vi "SetLightTower&Switch.vi"(6 "Supress Match Error (F)":bool, 8 "error in (no error)":errorcluster, 9 "UpdateValue? (F)":bool[](array[boolean]), 10 "RoomAlert Device":T1, 11 "RoomAlert in":refnum<class "RoomAlert.lvclass">) -> (0 "error out":errorcluster, 3 "RoomAlert out":refnum<class "RoomAlert.lvclass">)   [LabVIEW 2018, in "SensorPlugins.lvlib" / "RoomAlert.lvclass"]
doc: "Sets the LED and audio value of the LightTower alarm."
uses:
  RoomAlert.lvclass
  TypeDefinitions/RoomAlertControls.ctl
  RoomAlert.lvclass/RoomAlert.ctl
  <vilib>/Utility/error.llb/Error Cluster From Error Code.vi
  <vilib>/ErrorRing/Error Ring.xnode
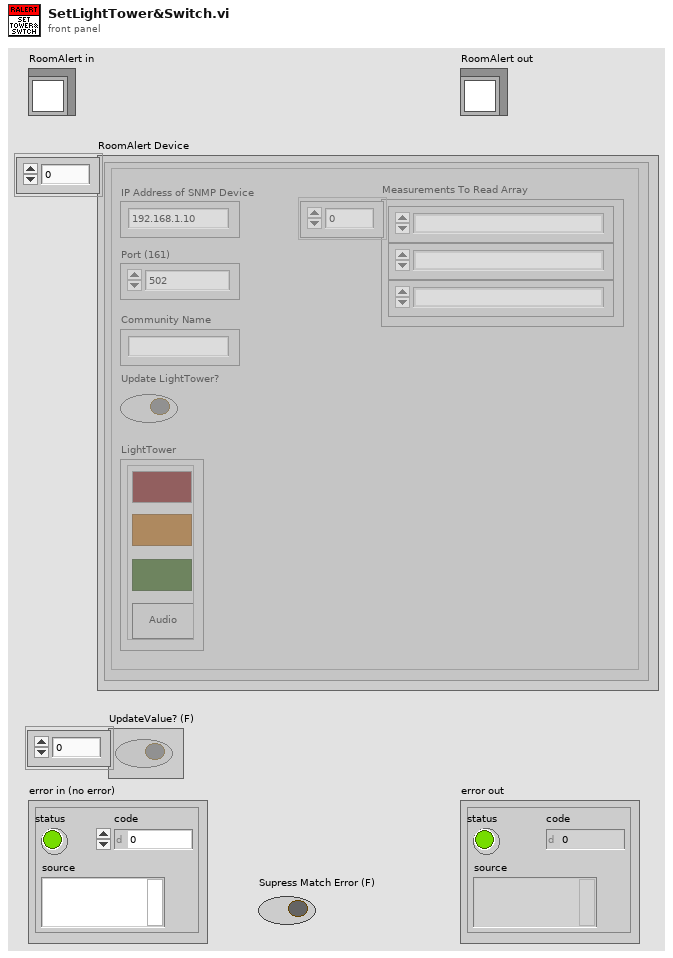
[diagram p1: front panel]
types:
  T1 = typedef "SensorPlugins.lvlib/RoomAlert.lvclass/RoomAlertControls.ctl" = cluster{"Connected?":bool, "IP Address of SNMP Device":string, "Port (161)":u16, "Community Name":string, "Measurements To Read Array":u16[], "Update LightTower?":bool, "LightTower":cluster{"Red":bool, "Amber":bool, "Green":bool, "Audio":bool}, "RoomAlert Model ID":string, "Sensor OID Numbers":string[][], "Sensor Light Tower OID Numbers":string[][]}[]
  T2 = typedef "SensorPlugins.lvlib/RoomAlert.lvclass/MeasurementControls.ctl" = cluster{"Measurement RefreshTime (ms)":u32, "Measurement Name":string, "Timeout(ms)":i32, "Amber Warning Light Configuration":cluster{"Warning Temperture (Degrees C)":dbl, "Temperature Delta (Degrees C/Minute)":dbl, "Time Window (Minutes)":dbl}}
  T3 = cluster{"Red":bool, "Amber":bool, "Green":bool, "Audio":bool}
  T4 = typedef "SensorPlugins.lvlib/RoomAlert.lvclass/CommunicationControls.ctl" = refnum<k16>[]
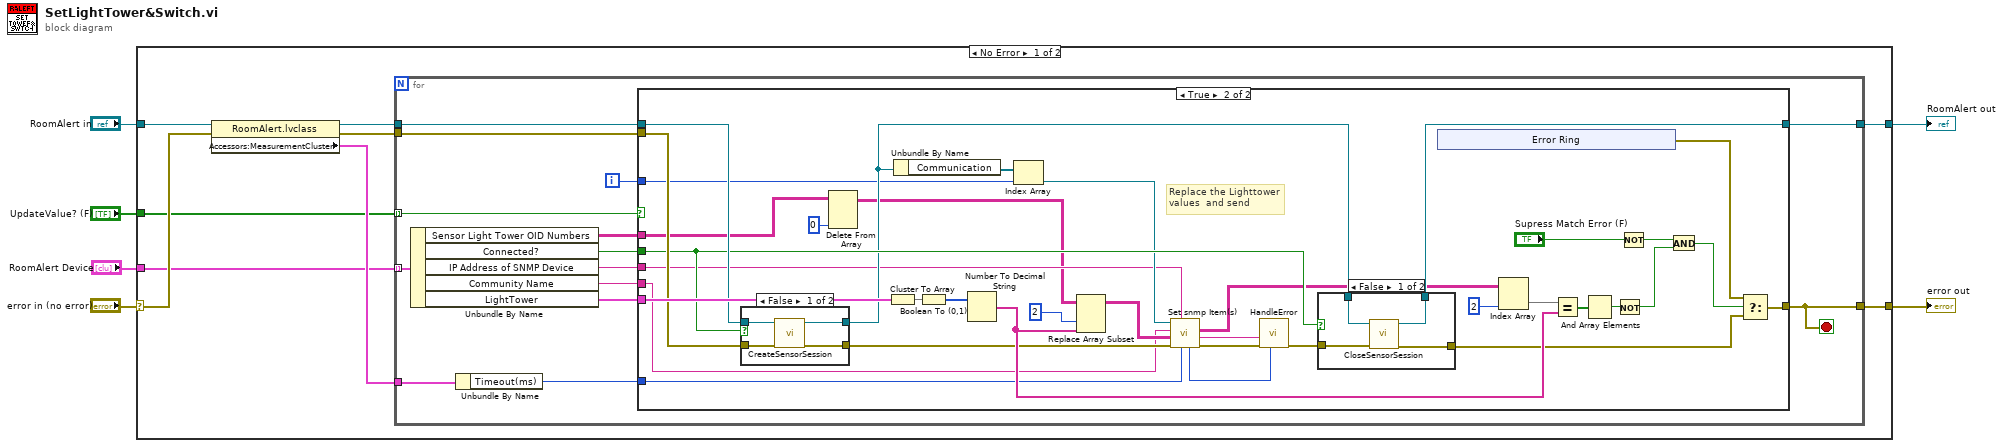
[diagram p0: block diagram]
diagram:
  n1 = case shown="No Error" "error in (no error)" {
    selector: "error in (no error)" -> [w14 w87]
    tunnel: [w12 w87] -> w5
    tunnel: [w10 w86] -> w3
    tunnel: "RoomAlert in" -> [w15 w86]
    tunnel: "RoomAlert Device" -> [w8 _]
    tunnel: "UpdateValue? (F)" -> [w7 _]
    frame No Error {
      n2 = property class="RoomAlert.lvclass"(reference=w15, error in=w14) -> (reference out=w11:refnum<class "RoomAlert.lvclass">, error out=w13:errorcluster, "Accessors:MeasurementCluster"=w9:T2)
      n3 = for {
        tunnel: w8 -> [w29] mode=indexing
        tunnel: w13 -> [w20]
        tunnel: [w25] -> w12
        tunnel: w11 -> [w22]
        tunnel: [w21] -> w10
        tunnel: w9 -> [w24]
        tunnel: w7 -> [w18] mode=indexing
        i -> [w17]
        stop <- w25 stop-if-true
        n4 = Unbundle By Name(w29) -> ("Sensor Light Tower OID Numbers"=w16:string[][], "Connected?"=w19:bool, "IP Address of SNMP Device"=w26:string, "Community Name"=w27:string, "LightTower"=w28:T3)
        n5 = Unbundle By Name(w24) -> ("Timeout(ms)"=w23:i32)
        n6 = case shown="True" w18 {
          tunnel: w28 -> [_ w68]
          tunnel: w27 -> [_ w40]
          tunnel: w26 -> [_ w41]
          tunnel: [w30 w67] -> w25
          tunnel: w23 -> [_ w45]
          tunnel: w22 -> [w31 w53]
          tunnel: [w31 w55] -> w21
          tunnel: w20 -> [w30 w54]
          tunnel: w19 -> [_ w52]
          tunnel: w17 -> [_ w49]
          tunnel: w16 -> [_ w34]
          frame False {
          }
          frame True {
            # "Replace the Lighttower\nvalues  and send"
            n7 = case shown="False" w52 {
              tunnel: w54 -> [w72 w74]
              tunnel: [w71 w74] -> w48
              tunnel: w53 -> [w70 w73]
              tunnel: [w69 w73] -> w51
              frame False {
                n8 = call-dynamic "CreateSensorSession.vi"("error in (no error)"=w72, "RoomAlert in"=w70) -> ("error out"=w71:errorcluster, "RoomAlert out"=w69:refnum<class "RoomAlert.lvclass">)  [unwired: 8 in]
              }
              frame True {
              }
            }
            n9 = Delete From Array(array=w34, index (col)=0 ("disabled index (col)")) -> (array with subset deleted=w32:string[][])  [unwired: 2 in, 1 out]
            n10 = Cluster To Array(cluster=w68) -> (array=w66:bool[])
            n11 = Unbundle By Name(w51) -> ("Communication"=w50:T4)
            n12 = Boolean To (0,1)(Boolean=w66) -> (0, 1=w65:i16[])
            n13 = Number To Decimal String(number=w65) -> (decimal integer string=w63:string[])  [unwired: 1 in]
            n14 = Index Array(array=w50, index=w49) -> (element=w43:refnum<k16>)
            n15 = Replace Array Subset(array=w32, new element=w63, index (col)=2 ("disabled index (col)")) -> (w42:string[][])  [unwired: 1 in]
            n16 = call "Set snmp Item(s).vi"("timeout ms (25000)"=w45, "IP Address of SNMP Device"=w41, "error in (no error)"=w48, "OID/TYPE/VALUE ARRAY"=w42, "Community Name"=w40, "connection ID in"=w43) -> ("error out"=w47:errorcluster, "error-string"=w46:string, "SnmpDataAsStrings"=w35:string[][], "error-status"=w44:u8)  [unwired: 2 out]
            n17 = call "HandleError.vi"("error-status"=w44, "Error In"=w47, "Error String"=w46) -> ("Error Out"=w57:errorcluster)  [unwired: 8 in]
            n18 = case shown="False" w52 {
              tunnel: w57 -> [w78 w79]
              tunnel: [w77 w79] -> w56
              tunnel: [w76 w80] -> w55
              tunnel: w51 -> [w75 w80]
              frame False {
                n19 = call-dynamic "CloseSensorSession.vi"("error in (no error)"=w78, "RoomAlert in"=w75) -> ("error out"=w77:errorcluster, "RoomAlert out"=w76:refnum<class "RoomAlert.lvclass">)  [unwired: 8 in]
              }
              frame True {
              }
            }
            n20 = xnode "Error Ring"() -> ("error out"=w58:errorcluster)
            n21 = Index Array(array=w35, index (col)=2 ("disabled index (col)")) -> (element=w61:string[])  [unwired: 1 in]
            n22 = Equal?(x=w61, y=w63) -> (x = y?=w60:bool[])
            n23 = And Array Elements(Boolean array=w60) -> (logical AND=w59:bool)
            n24 = Not(x=w59) -> (.not. x?=w37:bool)
            n25 = Not(x="Supress Match Error (F)") -> (.not. x?=w38:bool)
            n26 = And(x=w38, y=w37) -> (x .and. y?=w36:bool)
            n27 = Select(t=w58, s=w36, f=w56) -> (s? t:f=w67:errorcluster)
          }
        }
      }
    }
    frame Error {
    }
  }
  "error out" <- w5
  "RoomAlert out" <- w3
